vi "Read Config Version.vi"(8 "error in (no error)":errorcluster, 11 "Sequence Config in":refnum<class "Sequence Config.lvclass">) -> (0 "error out":errorcluster, 2 "String":string, 3 "Sequence Config out":refnum<class "Sequence Config.lvclass">)   [LabVIEW 2015, in "Sequence Config.lvclass"]
uses:
  Sequence Config.lvclass
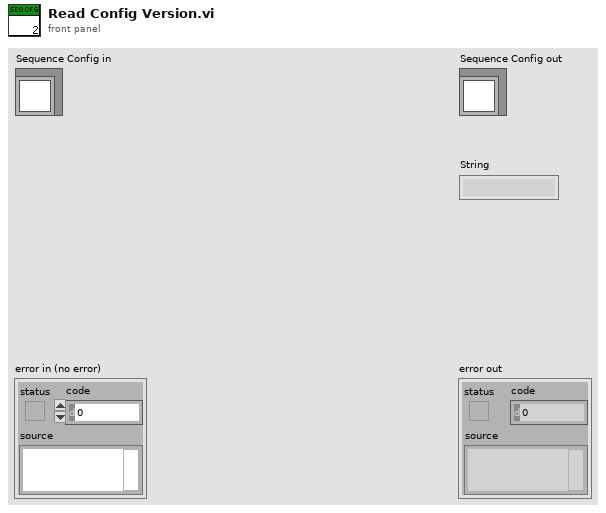
[diagram p1: front panel]
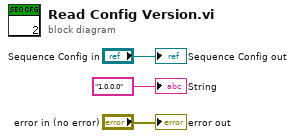
[diagram p0: block diagram]
diagram:
  "error out" <- "error in (no error)"
  "Sequence Config out" <- "Sequence Config in"
  "String" <- "1.0.0.0" ("String")
